vi "Retrieve Encoded Name.vi"(11 "TCP Network Connection in":refnum<k5>) -> (0 "bytes consumed":u32, 2 "Name":string, 3 "TCP Network Connection in 2":refnum<k5>)   [LabVIEW 2017]
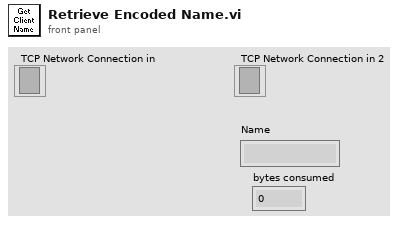
[diagram p1: front panel]
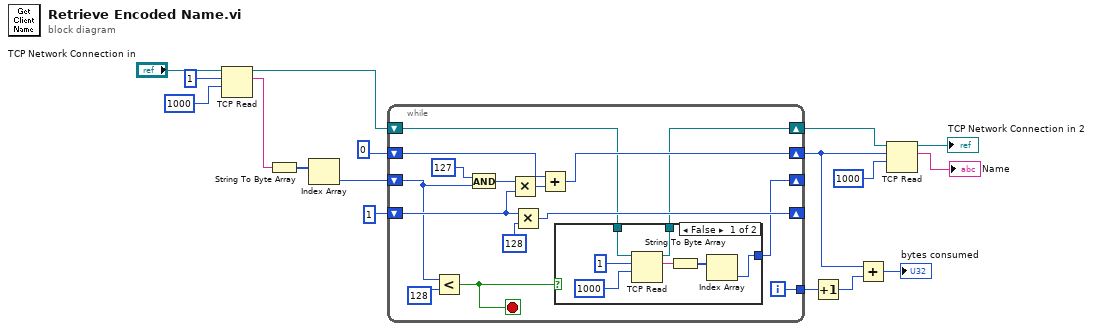
[diagram p0: block diagram]
diagram:
  n1 = TCP Read(connection ID="TCP Network Connection in", bytes to read=1, 9:1000 ("timeout ms (25000)")) -> (connection ID out=w8:refnum<k5>, data out=w11:string)  [unwired: 2 in, 1 out]
  n2 = String To Byte Array(string=w11) -> (unsigned byte array=w10:u8[])
  n3 = Index Array(array=w10) -> (element=w9:u8)  [unwired: 1 in]
  n4 = while {
    shift-right: [w31] -> w3
    shift-left: u32 0 -> [w32]
    shift-right: [w29] -> _
    shift-left: u32 1 -> [w30]
    tunnel: [w23] -> w12
    shift-right: [w20] -> _
    shift-left: w9 -> [w22]
    shift-right: [w18] -> w6
    shift-left: w8 -> [w19]
    i -> [w23]
    stop <- w21 stop-if-true
    n5 = Less?(x=w22, y=u32 128) -> (x < y?=w21:bool)
    n6 = And(x=u8 127, y=w22) -> (x .and. y?=w25:u8)
    n7 = Multiply(x=w25, y=w30) -> (x*y=w27:u32)
    n8 = Multiply(x=w30, y=u32 128) -> (x*y=w29:u32)
    n9 = Add(x=w32, y=w27) -> (x+y=w31:u32)
    n10 = case shown="False" w21 {
      tunnel: [w35 _] -> w20
      tunnel: w19 -> [w34 w40]
      tunnel: [w33 w40] -> w18
      frame False {
        n11 = TCP Read(connection ID=w34, bytes to read=1, 9:1000 ("timeout ms (25000)")) -> (connection ID out=w33:refnum<k5>, data out=w36:string)  [unwired: 2 in, 1 out]
        n12 = String To Byte Array(string=w36) -> (unsigned byte array=w37:u8[])
        n13 = Index Array(array=w37) -> (element=w35:u8)  [unwired: 1 in]
      }
      frame True {
      }
    }
  }
  n14 = Increment(x=w12) -> (x+1=w2:i32)
  n15 = Add(x=w3, y=w2) -> (x+y=→"bytes consumed":u32)
  n16 = TCP Read(connection ID=w6, bytes to read=w3, 9:1000 ("timeout ms (25000)")) -> (connection ID out=→"TCP Network Connection in 2":refnum<k5>, data out=→"Name":string)  [unwired: 2 in, 1 out]
